vi "Filtration.vi"(5 "order":i32, 6 "Pulse/Resolution":i32, 7 "low cutoff freq [Hz]":dbl, 8 "error in (no error)":errorcluster, 9 "Tacho in":waveform(dbl)[](array[waveform]), 10 "Data in":waveform(dbl)[](array[waveform]), 11 "Sample rate":i64) -> (0 "error out":errorcluster, 1 "Data out":waveform(dbl)[][](array[waveform]), 3 "speed [rpm]":dbl, 4 "Tacho out":waveform(dbl))   [LabVIEW 2021]
uses:
  <vilib>/addons/Digital Filter Design/Process.llb/DFD Filtering (Wfm NChan).vi
  <vilib>/addons/Sound and Vibration/Order Analysis/Tach Process/OAT Analog Tacho Process (1 Tacho).vi
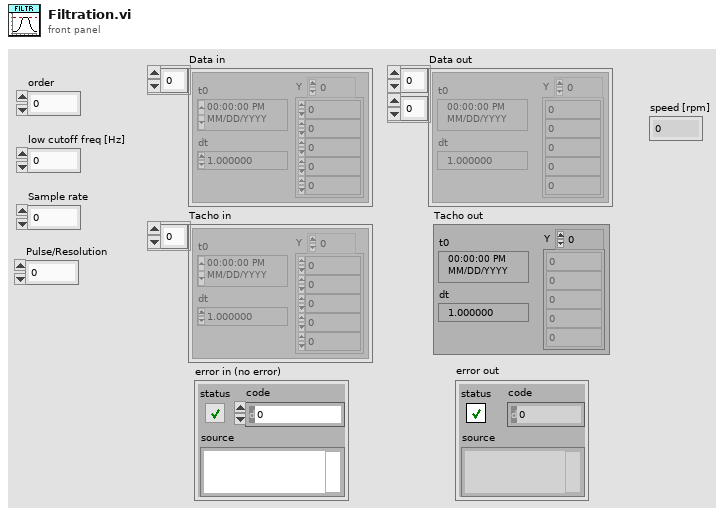
[diagram p1: front panel]
types:
  T1 = enum16{"Lowpass", "Highpass", "Bandpass", "Bandstop"}
  T2 = typedef "NI_DigFilterLicensed.lvlib/DFD Filter Obj.ctl" = cluster{"mSRate_Fs":dbl, "mSRate_Version":string, "mSRate_Comments":string, "mSRate_OrgCoef":T3, "mSRate_CurCoef":T3, "mSRate_Quantized?":bool, "mSRate_QCoef":T3, "mSRate_QSettings":T5[], "mSRate_Order":i32, "mSRate_Scaling":cluster{"mSRate_ScaleByPowerOf2?":bool, "mSRate_ScaleType":T7}}
  T3 = typedef "NI_DigFilterLicensed.lvlib/DFD Filter Coef.ctl" = cluster{"type":T4, "gain":dbl, "coef a (k)":dbl[], "coef b (v)":dbl[]}
  T4 = typedef "NI_DigFilterLicensed.lvlib/DFD Filter Structure Type Selector.ctl" = enum16{"Undefined", "FIR Direct Form", "FIR Direct Form Transposed", "FIR Symmetric", "FIR Antisymmetric", "IIR Direct Form I", "IIR Direct Form I Transposed", "IIR Direct Form II", "IIR Direct Form II Transposed", "IIR Cascaded Second Order Sections Form I", "IIR Cascaded Second Order Sections Form I Transposed", "IIR Cascaded Second Order Sections Form II", "IIR Cascaded Second Order Sections Form II Transposed", "Lattice Allpass (basic sections)", "Lattice Allpass (one multiplier sections)", "Lattice Allpass (normalized sections)", "Lattice AR (basic sections)", "Lattice AR (one multiplier sections)", "Lattice AR (normalized sections)", "Lattice MA (minimum phase)", "Lattice MA (maximum phase)", "Lattice ARMA (basic sections)", "Lattice ARMA (one multiplier sections)", "Lattice ARMA (normalized sections)"}
  T5 = typedef "NI_DigFilterLicensed.lvlib/dfd_Internal Quantization Settings.ctl" = cluster{"source":T6, "wl":i16, "iwl":i16, "overflow mode":enum16{"Saturation", "Wrap"}, "rounding mode":enum16{"Nearest", "Truncation"}, "signed?":bool}
  T6 = typedef "NI_DigFilterLicensed.lvlib/dfd_Internal Quantization Srcs.ctl" = u16
  T7 = typedef "NI_DigFilterLicensed.lvlib/DFD Coef Norm Type.ctl" = enum16{"No Norm", "Time Domain 1-Norm", "Time Domain 2-Norm", "Time Domain Inf-Norm"}
  T8 = typedef "SoundVib_TachProcess.lvlib/speed profile.ctl" = cluster{"time [s]":dbl[], "speed [RPM]":dbl[]}
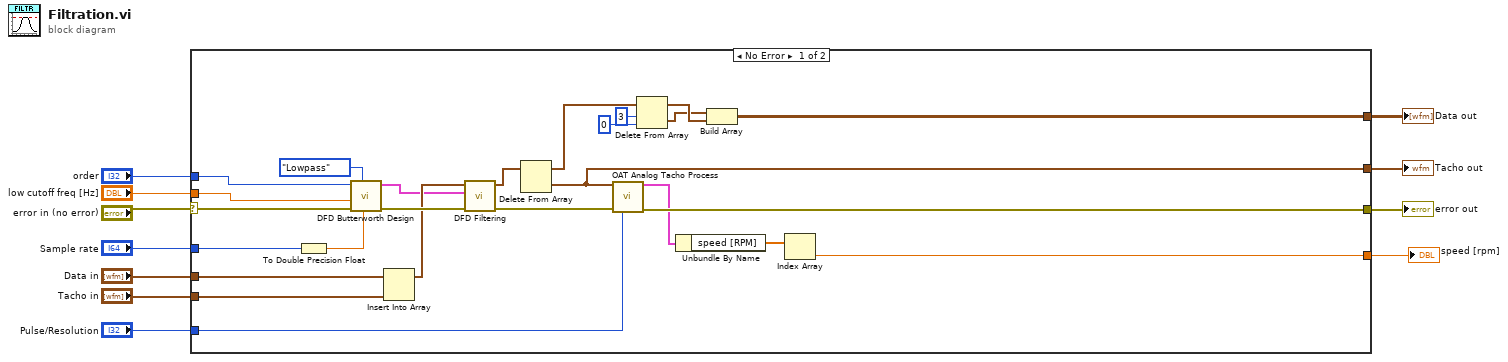
[diagram p0: block diagram]
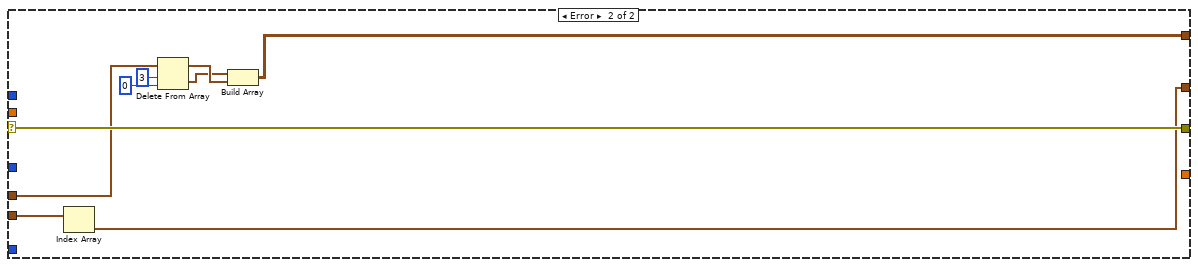
[diagram p2: hidden frame]
diagram:
  n1 = case shown="No Error" "error in (no error)" {
    selector: "error in (no error)" -> [w22 w45]
    tunnel: [w36 w45] -> w11
    tunnel: [w35 w37] -> w10
    tunnel: "Pulse/Resolution" -> [w28 _]
    tunnel: "low cutoff freq [Hz]" -> [w13 _]
    tunnel: "Sample rate" -> [w15 _]
    tunnel: "Tacho in" -> [w24 w44]
    tunnel: "Data in" -> [w23 w38]
    tunnel: "order" -> [w20 _]
    tunnel: [w16 w43] -> w2
    tunnel: [w12 _] -> w1
    frame No Error {
      n2 = To Double Precision Float(number=w15) -> (double precision float=w14:dbl)
      n3 = call <vilib>:"DFD Butterworth Design.vi"("fs [Hz]"=w14, "filter type"=T1."Lowpass", "error in (no error)"=w22, "low cutoff freq [Hz]"=w13, "order"=w20) -> ("error out"=w26:errorcluster, "filter out"=w19:T2)  [unwired: 5 in]
      n4 = Insert Into Array(array=w23, new element=w24) -> (w25:waveform(dbl)[])  [unwired: 1 in]
      n5 = call-poly <vilib>:"DFD Filtering.vi"("error in (no error)"=w26, "filter"=w19, "signal in"=w25) -> ("error out"=w27:errorcluster, "signal out"=w29:waveform(dbl)[])  [unwired: 7 in]
      n6 = Delete From Array(array=w29) -> (deleted portion=w16:waveform(dbl), array with subset deleted=w17:waveform(dbl)[])  [unwired: 2 in]
      n7 = call-poly <vilib>:"OAT Analog Tacho Process.vi"("analog tacho signal"=w16, "error in (no error)"=w27, "pulse width (2)"=w28) -> ("speed profile"=w30:T8, "error out"=w36:errorcluster)  [unwired: 8 in, 3 out]
      n8 = Delete From Array(array=w17, length=3, index=0) -> (deleted portion=w33:waveform(dbl)[], array with subset deleted=w34:waveform(dbl)[])
      n9 = Unbundle By Name(w30) -> ("speed [RPM]"=w18:dbl[])
      n10 = Build Array(w33, w34) -> (w35:waveform(dbl)[][])
      n11 = Index Array(array=w18) -> (element=w12:dbl)  [unwired: 1 in]
    }
    frame Error {
      n12 = Index Array(array=w44) -> (element=w43:waveform(dbl))  [unwired: 1 in]
      n13 = Delete From Array(array=w38, length=3, index=0) -> (deleted portion=w41:waveform(dbl)[], array with subset deleted=w42:waveform(dbl)[])
      n14 = Build Array(w41, w42) -> (w37:waveform(dbl)[][])
    }
  }
  "Data out" <- w10
  "error out" <- w11
  "Tacho out" <- w2
  "speed [rpm]" <- w1
